vi "complete integration (1) (1).vi"() -> ()   [LabVIEW 2017]
uses:
  <vilib>/measure/NI_MABase.lvlib
panel:
  in  "signal type 4":T1(ring)
  in  "frequency 4":dbl=10.0 format="%0.2p"
  in  "signal type 3":T1(ring)
  in  "frequency 3":dbl=10.0 format="%0.2p"
  out "Flame voltage":dbl
  out "mq6 voltage":dbl
  out "Waveform Chart":dynamicdata(graph)
  out "Low Lighing":bool
  out "High Temperature":bool
  out "Low Temperature":bool
  out "Thermometer":dbl(slide) scale=0.0..50.0
  out "LDR Output (V)":dbl
  out "Temperatue (C)":dbl
  out "Temperature in (mV)":dbl
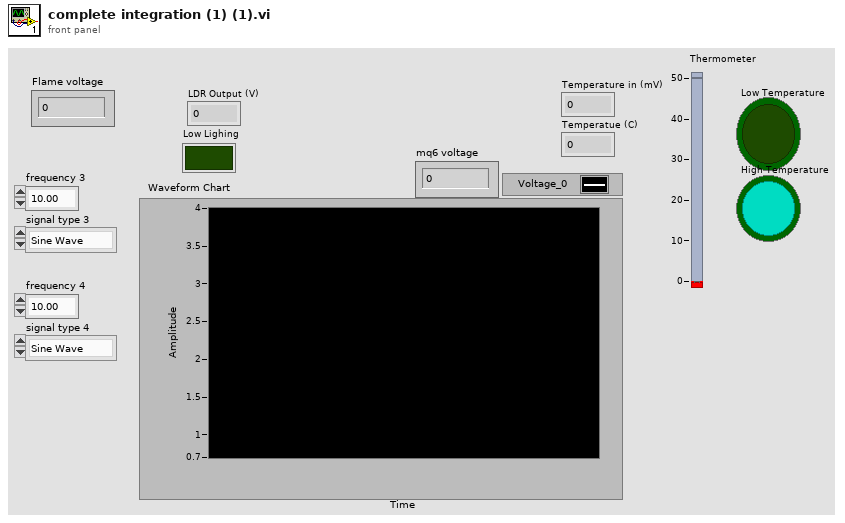
[diagram p1: front panel]
types:
  T1 = enum16{"Sine Wave", "Triangle Wave", "Square Wave", "Sawtooth Wave"}
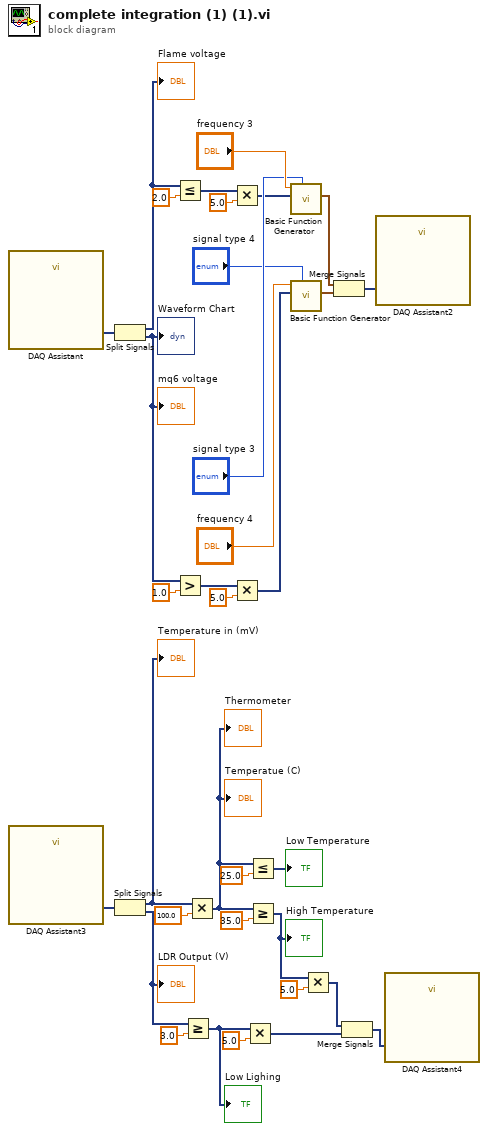
[diagram p0: block diagram]
diagram:
  n1 = call "DAQ Assistant"() -> ("data"=w6:dynamicdata)  [unwired: 16 in, 3 out]
  n2 = call "DAQ Assistant3"() -> ("data"=w22:dynamicdata)  [unwired: 16 in, 3 out]
  n3 = Split Signals(w6) -> (w18:dynamicdata, w2:dynamicdata)  [unwired: 2 in]
  "Waveform Chart" <- w2
  "mq6 voltage" <- w2
  "Flame voltage" <- w18
  n4 = Split Signals(w22) -> (w34:dynamicdata, w32:dynamicdata)  [unwired: 2 in]
  "Temperature in (mV)" <- w34
  "LDR Output (V)" <- w32
  n5 = Less Or Equal?(x=w18, y=2.0) -> (x <= y?=w13:dynamicdata)
  n6 = Greater?(x=w2, y=1.0) -> (0:w1:dynamicdata)
  n7 = Greater Or Equal?(x=w32, y=3.0) -> (x >= y?=w24:dynamicdata)
  "Low Lighing" <- w24
  n8 = Multiply(x=w34, y=100.0) -> (x*y=w27:dynamicdata)
  "Temperatue (C)" <- w27
  "Thermometer" <- w27
  n9 = Multiply(x=w13, y=5.0) -> (x*y=w11:dynamicdata)
  n10 = Multiply(x=w1, y=5.0) -> (x*y=w9:dynamicdata)
  n11 = Multiply(x=w24, y=5.0) -> (x*y=w4:dynamicdata)
  n12 = Less Or Equal?(x=w27, y=25.0) -> (x <= y?=→"Low Temperature":dynamicdata)
  n13 = Greater Or Equal?(x=w27, y=35.0) -> (x >= y?=w26:dynamicdata)
  "High Temperature" <- w26
  n14 = call <vilib>:"Basic Function Generator.vi"("signal type"="signal type 3", "amplitude"=w11, "frequency"="frequency 3") -> ("signal out"=w8:waveform(dbl))  [unwired: 6 in, 2 out]
  n15 = call <vilib>:"Basic Function Generator.vi"("signal type"="signal type 4", "amplitude"=w9, "frequency"="frequency 4") -> ("signal out"=w7:waveform(dbl))  [unwired: 6 in, 2 out]
  n16 = Multiply(x=w26, y=5.0) -> (x*y=w3:dynamicdata)
  n17 = Merge Signals(w8, w7) -> (w5:dynamicdata)
  n18 = Merge Signals(w3, w4) -> (w21:dynamicdata)
  n19 = call "DAQ Assistant2"("data"=w5) -> ()  [unwired: 16 in, 3 out]
  n20 = call "DAQ Assistant4"("data"=w21) -> ()  [unwired: 16 in, 3 out]
